vi "MAINP Update ECUs.vi"(6 "First?":bool, 7 "Controls":refnum<vi>[](array[refnum]), 8 "error in (no error)":errorcluster, 10 "Alias":string, 11 "Device Item Ref in":T1 format="%.0x") -> (0 "error out":errorcluster, 3 "Device Item Ref out":T1 format="%.0x")   [LabVIEW 2018, in "CAN Gateway System Explorer.lvlib"]
uses:
  CAN Gateway System Explorer.lvlib
  <vilib>/NI Veristand/Custom Device API/Custom Device Item Ref.ctl
  Shared/Constants.vi
  <vilib>/NI Veristand/Custom Device API/Get Item Property (String).vi
  <vilib>/NI Veristand/Custom Device API/Set Item Property (String).vi
  <vilib>/NI Veristand/Custom Device API/Custom Device API.lvlib
  Shared/CAN Gateway Shared.lvlib
  <resource>/objmgr/xnet.rc
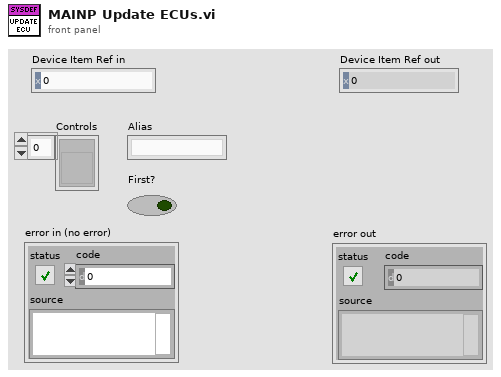
[diagram p1: front panel]
types:
  T1 = typedef "Custom Device API.lvlib/Custom Device Item Ref.ctl" = u64
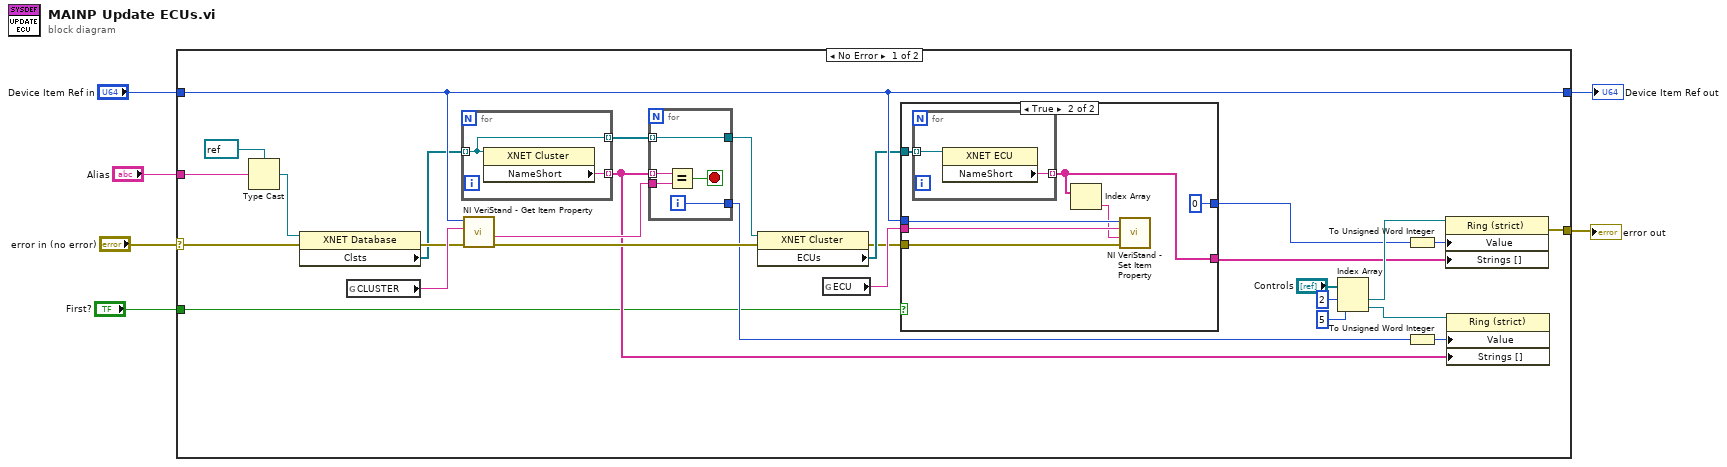
[diagram p0: block diagram]
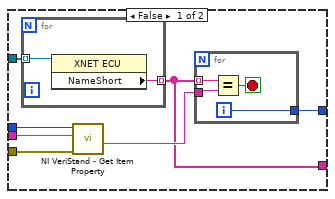
[diagram p2: hidden frame]
diagram:
  n1 = case shown="No Error" "error in (no error)" {
    selector: "error in (no error)" -> [w26 w65]
    tunnel: "Device Item Ref in" -> [w23 w64]
    tunnel: [w23 w64] -> w4
    tunnel: [w30 w65] -> w3
    tunnel: "Alias" -> [w27 _]
    tunnel: "First?" -> [w7 _]
    frame No Error {
      n2 = Type Cast(type=refnum<k21> refnum ("XNET Database"), x=w27) -> (*(type *) &x=w29:refnum<k21>)
      n3 = property class="XNET Database"(reference=w29, error in=w26) -> (error out=w24:errorcluster, "Clsts"=w22:refnum<k21>[])  [unwired: 1 out]
      n4 = global read "Constants.vi" "CLUSTER"() -> (w25:string)
      n5 = for {
        tunnel: w22 -> [w62] mode=indexing
        tunnel: [w63] -> w18 mode=indexing
        tunnel: [w62] -> w20 mode=indexing
        n6 = property class="XNET Cluster"(reference=w62) -> ("NameShort"=w63:string)  [unwired: 1 in, 2 out]
      }
      n7 = call-poly <vilib>:"NI VeriStand - Get Item Property.vi"("error in (no error)"=w24, "Property Name"=w25, "Item Ref in"=w23) -> ("error out"=w21:errorcluster, "Value"=w19:string)  [unwired: 5 in, 2 out]
      n8 = for {
        tunnel: [w60] -> w15
        tunnel: w18 -> [w59] mode=indexing
        tunnel: w20 -> [w57] mode=indexing
        tunnel: w19 -> [w58]
        tunnel: [w57] -> w17
        i -> [w60]
        stop <- w61 stop-if-true
        n9 = Equal?(x=w59, y=w58) -> (x = y?=w61:bool)
      }
      n10 = property class="XNET Cluster"(reference=w17, error in=w21) -> (error out=w13:errorcluster, "ECUs"=w14:refnum<k21>[])  [unwired: 1 out]
      n11 = global read "Constants.vi" "ECU"() -> (w32:string)
      n12 = case shown="True" w7 {
        tunnel: w32 -> [w41 w50]
        tunnel: w23 -> [w39 w51]
        tunnel: w14 -> [w38 w54]
        tunnel: w13 -> [w37 w52]
        tunnel: [w36 w49] -> w12
        tunnel: [w35 0] -> w11
        frame False {
          n13 = for {
            tunnel: w38 -> [w42] mode=indexing
            tunnel: [w43] -> w36 mode=indexing
            n14 = property class="XNET ECU"(reference=w42) -> ("NameShort"=w43:string)  [unwired: 1 in, 2 out]
          }
          n15 = call-poly <vilib>:"NI VeriStand - Get Item Property.vi"("error in (no error)"=w37, "Property Name"=w41, "Item Ref in"=w39) -> ("Value"=w40:string)  [unwired: 5 in, 3 out]
          n16 = for {
            tunnel: w40 -> [w47]
            tunnel: [w45] -> w35
            tunnel: w36 -> [w44] mode=indexing
            i -> [w45]
            stop <- w46 stop-if-true
            n17 = Equal?(x=w44, y=w47) -> (x = y?=w46:bool)
          }
        }
        frame True {
          n18 = for {
            tunnel: w54 -> [w55] mode=indexing
            tunnel: [w56] -> w49 mode=indexing
            n19 = property class="XNET ECU"(reference=w55) -> ("NameShort"=w56:string)  [unwired: 1 in, 2 out]
          }
          n20 = Index Array(array=w49) -> (element=w48:string)  [unwired: 1 in]
          n21 = call-poly <vilib>:"NI VeriStand - Set Item Property.vi"("error in (no error)"=w52, "Value"=w48, "Property Name"=w50, "Item Ref in"=w51) -> ()  [unwired: 5 in, 3 out]
        }
      }
      n22 = Index Array(array="Controls", index #1=2 ("index"), index #2=5 ("index")) -> (element #1=w31:refnum<vi>, element #2=w8:refnum<vi>)
      n23 = To Unsigned Word Integer(number=w11) -> (unsigned 16bit integer=w10:u16)
      n24 = To Unsigned Word Integer(number=w15) -> (unsigned 16bit integer=w16:u16)
      n25 = property class="Ring (strict)"(reference=w31, "Value"=w10, "Strings []"=w12) -> (error out=w30:errorcluster)  [unwired: 1 in, 1 out]
      n26 = property class="Ring (strict)"(reference=w8, "Value"=w16, "Strings []"=w18) -> ()  [unwired: 1 in, 2 out]
    }
    frame Error {
    }
  }
  "error out" <- w3
  "Device Item Ref out" <- w4
